vi "Main LOER Signal Example.vi"() -> ()   [LabVIEW 2016]
uses:
  SignalWithAlarm Class/SignalWithAlarm.lvclass/SignalWithAlarm.ctl
  SignalWithAlarm Class/Read LimitOverride.vi
  <extravilib>/ChannelInstances/Tag-bool/Read With Abort.vi
  <extravilib>/ChannelInstances/Tag-bool/Write With Abort.vi
  <extravilib>/ChannelInstances/Tag-bool/Instantiate.vi
  <extravilib>/ChannelInstances/Tag-bool/EndpointRead.vi
  <extravilib>/ChannelInstances/Tag-bool/Endpoint.vi
  <vilib>/LOER/LOER XNode/LV Object Event Registration Node.xnode
  SignalWithAlarm Class/SignalWithAlarm.lvclass
  <extravilib>/ChannelInstances/Tag-bool.lvlib
panel:
  out "Latest Limit Override Value":dbl caption="Numeric"
  out "Signal":dbl(graph) caption="Waveform Chart"
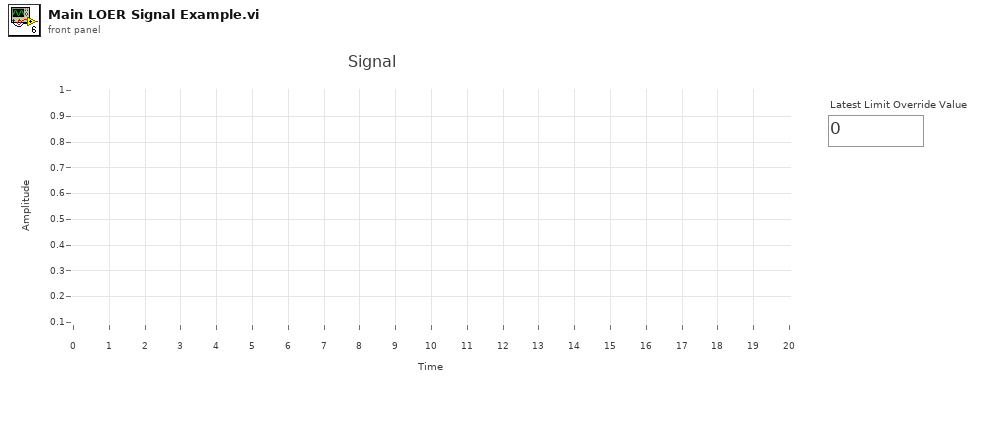
[diagram p1: front panel]
types:
  T1 = typedef "Tag-bool.lvlib/))Channel.ctl" = refnum<queue>
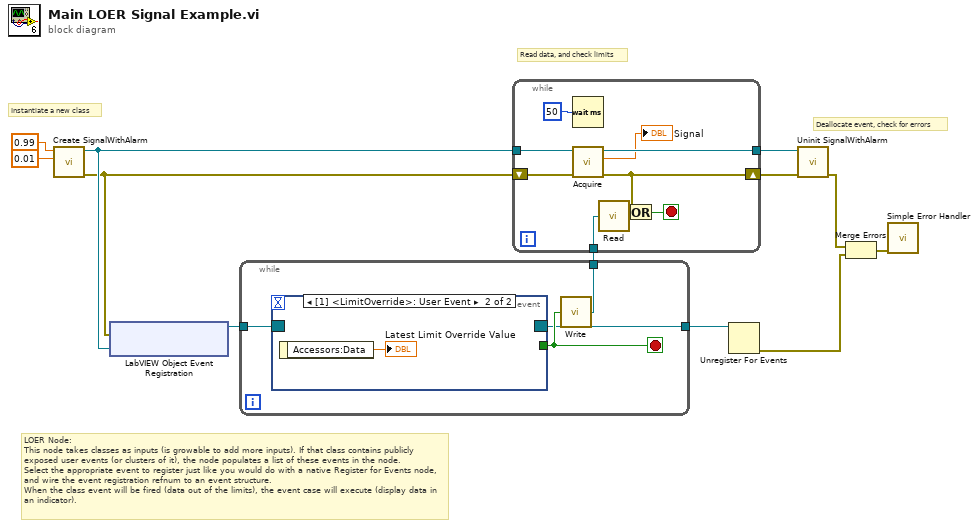
[diagram p0: block diagram]
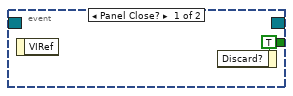
[diagram p2: hidden frame]
diagram:
  # "Deallocate event, check for errors"
  # "Read data, and check limits"
  # "LOER Node:\nThis node takes classes as inputs (is growable to add more inputs). If that class contains publicly exposed user events (or clusters of it), the node populates a list of these events in the node.\nSelect the appropriate event to register just like you would do with a native Register for Events node, and wire the event registration refnum to an event structure.\nWhen the class event will be fired (data out of the limits), the event case will execute (display data in an indicator)."
  # "Instantiate a new class"
  n1 = call "Create SignalWithAlarm.vi"("Low Limit"=0.01, "High Limit"=0.99) -> ("error out"=w10:errorcluster, "SignalWithAlarm out"=w12:refnum<class "SignalWithAlarm.lvclass">)  [unwired: 8 in]
  n2 = xnode "LabVIEW Object Event Registration"("Error In"=w10, "Object_1"=w12) -> ("Event Registration Refnum"=w11:refnum<event-registration>)  [unwired: 1 out]
  n3 = while {
    tunnel: w11 -> [w15]
    tunnel: [w14] -> w9
    tunnel: [w13] -> w8
    stop <- w16 stop-if-true
    n4 = event shown="[1] <LimitOverride>: User Event" {
      selector: w15 -> [_ _]
      dyn-events: [_ _] -> w14
      timeout: _ -> [_ _]
      tunnel: [w17 _] -> w16
      event Panel Close? {
        w17 = TRUE ("Discard?")
        n5 = event-data() -> ()  [unwired: 1 in, 1 out]
        n6 = event-data("Discard?"=w17) -> ()  [unwired: 1 in, 1 out]
      }
      event User Event {
        n7 = event-data() -> ("Accessors:Data"=→"Latest Limit Override Value":dbl)  [unwired: 1 in]
      }
    }
    n8 = call <extravilib>:"Write.vi"("element"=w16) -> ("channel"=w13:T1)  [unwired: 1 out]
  }
  n9 = while {
    tunnel: w12 -> [w27]
    shift-right: [w23] -> w5
    shift-left: w10 -> [w26]
    tunnel: w8 -> [w24]
    tunnel: [w20] -> w7
    stop <- w21 stop-if-true
    n10 = Wait (ms)(milliseconds to wait=u32 50) -> ()  [unwired: 1 out]
    n11 = call-dynamic "Acquire.vi"("error in (no error)"=w26, "SignalWithAlarm in"=w27) -> ("error out"=w23:errorcluster, "Data"=→"Signal":dbl, "SignalWithAlarm out"=w20:refnum<class "SignalWithAlarm.lvclass">)  [unwired: 7 in]
    n12 = call <extravilib>:"Read.vi"("channel"=w24) -> ("element"=w22:bool)  [unwired: 1 in, 1 out]
    n13 = Or(x=w23, y=w22) -> (x .or. y?=w21:bool)
  }
  n14 = Unregister For Events(event registration refnum=w9) -> (error out=w3:errorcluster)  [unwired: 1 in]
  n15 = call "Uninit SignalWithAlarm.vi"("error in (no error)"=w5, "SignalWithAlarm in"=w7) -> ("error out"=w4:errorcluster)  [unwired: 8 in, 1 out]
  n16 = Merge Errors(w4, w3) -> (w6:errorcluster)
  n17 = call <vilib>:"Simple Error Handler.vi"("error in (no error)"=w6) -> ()  [unwired: 4 in, 5 out]
